vi "Test Namer WIth Shared Approval File Default Behavior.vi"(11 "Test Case In":refnum<class "Namer Tests.lvclass">) -> (0 "error out":errorcluster, 3 "Test Case Out":refnum<class "Namer Tests.lvclass">)   [LabVIEW 2020, in "Namer Tests.lvclass"]
uses:
  Namer Tests.lvclass
  C:/Program Files/National Instruments/LabVIEW 2026/vi.lib/Astemes/LUnit/Test Case.lvclass
  Source/Approval Tests/Namer With Shared Approved File/Namer With Shared Approved File.lvclass
  Source/Approval Tests/Naming Data/Naming Data.lvclass
  Source/Approval Tests/Naming Data/Naming Data.lvclass/Naming Data.ctl
  Source/Approval Tests/Namer With Shared Approved File/Namer With Shared Approved File.lvclass/Namer With Shared Approved File.ctl
  <vilib>/Astemes/LUnit/Test Case.lvclass/Test Case.ctl
  4993e8ee-a06a-463a-9684-69129f64d5ce.vi
  00e75abf-9e6d-40d3-bb97-1797755a17b4.vi
  Source/Approval Tests/Naming Data/Write Test VI Name.vi
  Source/Approval Tests/Naming Data/Write Extension.vi
  Source/Approval Tests/Naming Data/Write Test Label.vi
  Source/Approval Tests/Namer With Shared Approved File/Write Shared Approved File Path.vi
  <vilib>/Astemes/LUnit/Core/LUnit Test Case/Private/Append Pass Result.vi
  <vilib>/Astemes/LUnit/Core/LUnit Test Case/Private/Append Fail Result.vi
  4993e8ee-a06a-463a-9684-69129f64d5ce.vi/9c5d11cd-9439-4240-a1ee-d9baace9c924.vi
  00e75abf-9e6d-40d3-bb97-1797755a17b4.vi/9c5d11cd-9439-4240-a1ee-d9baace9c924.vi
  <vilib>/Astemes/LUnit/Core/LUnit Test Case/Private/Run In UI.vi
  <vilib>/Utility/error.llb/Clear Errors.vi
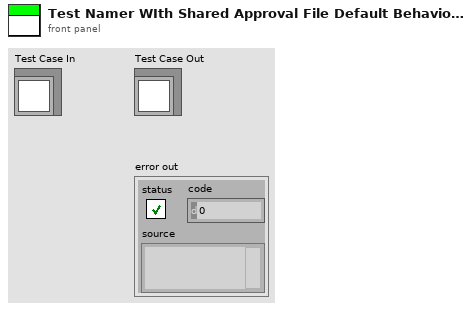
[diagram p1: front panel]
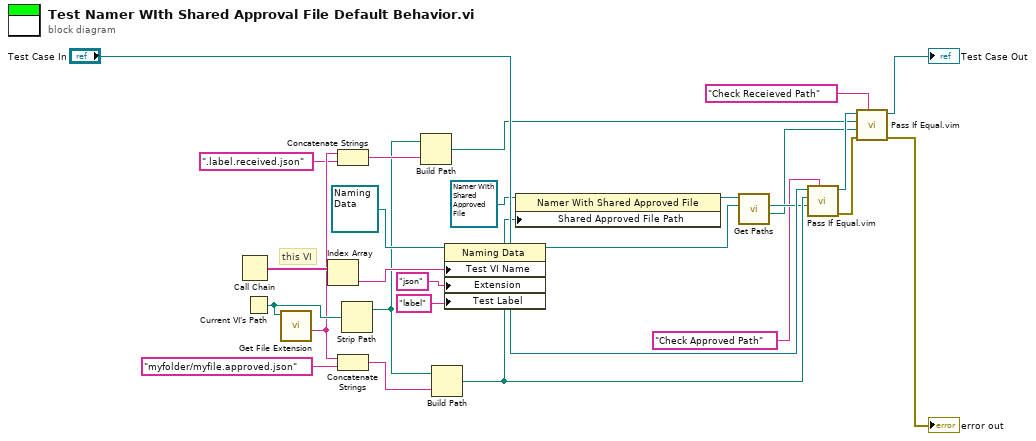
[diagram p0: block diagram]
diagram:
  # "this VI"
  n1 = Call Chain() -> (call chain=w21:string[])
  n2 = Current VI's Path() -> (path=w18:path)
  n3 = call <vilib>:"Get File Extension.vi"("file"=w18) -> ("filename without extension"=w17:string)  [unwired: 6 in, 4 out]
  n4 = Index Array(array=w21) -> (element=w20:string)  [unwired: 1 in]
  n5 = Concatenate Strings(w17, ".label.received.json" ("string")) -> (w14:string)
  n6 = Concatenate Strings(w17, "myfolder/myfile.approved.json" ("string")) -> (w13:string)
  n7 = Strip Path(path=w18) -> (stripped path=w10:path)  [unwired: 1 out]
  n8 = Build Path(base path=w10, name or relative path=w14) -> (appended path=w3:path)
  n9 = Build Path(base path=w10, name or relative path=w13) -> (appended path=w8:path)
  n10 = property on="Property Node" class="Naming Data"(reference=refnum<class "Naming Data.lvclass"> refnum ("Naming Data"), "Test VI Name"=w20, "Extension"="json", "Test Label"="label") -> (reference out=w19:refnum<class "Naming Data.lvclass">)  [unwired: 1 in, 1 out]
  n11 = property class="Namer With Shared Approved File"(reference=refnum<class "Namer With Shared Approved File.lvclass"> refnum ("Approval Tests:Namer with SubFolder.lvclass"), "Shared Approved File Path"=w8) -> (reference out=w9:refnum<class "Namer With Shared Approved File.lvclass">)  [unwired: 1 in, 1 out]
  n12 = call-dynamic "Get Paths.vi"("Naming Data"=w19, "Namer With Shared Approved File in"=w9) -> ("Received Path"=w2:path, "Approved Path"=w7:path)  [unwired: 6 in, 2 out]
  n13 = call "Pass If Equal.vim"("Description"="Check Approved Path" ("Label (VI Title)"), "Actual"=w7, "Expected"=w8, "LUnit Test Case In"="Test Case In") -> ("error out"=w25:errorcluster, "LUnit Test Case Out"=w5:refnum<class "Namer Tests.lvclass">)  [unwired: 6 in]
  n14 = call "Pass If Equal.vim"("Description"="Check Receieved Path" ("Label (VI Title)"), "error in (no error)"=w25, "Actual"=w2, "Expected"=w3, "LUnit Test Case In"=w5) -> ("error out"=→"error out":errorcluster, "LUnit Test Case Out"=→"Test Case Out":refnum<class "Namer Tests.lvclass">)  [unwired: 5 in]
